vi "Create Resources.vi"(0 "io resources":T1={"address"="SRAM\\Address", "read"="SRAM\\Read", "input valid"="SRAM\\Input Valid", "write data"="SRAM\\Write Data", "read data"="SRAM\\Read Data", "read data valid"="SRAM\\Read Data Valid", "ready for input"="SRAM\\Ready for Input"}) -> (4 "sram resources":T2={"io resources"={"address"="SRAM\\Address", "read"="SRAM\\Read", "input valid"="SRAM\\Input Valid", "write data"="SRAM\\Write Data", "read data"="SRAM\\Read Data", "read data valid"="SRAM\\Read Data Valid", "ready for input"="SRAM\\Ready for Input"}})   [LabVIEW 2011, in "niRFRIO SRAM 1.0.0 FPGA.lvlib"]
uses:
  <instrlib>/RF-RIO/SRAM/1.0.0/FPGA/niRFRIO SRAM 1.0.0 FPGA.lvlib
  <instrlib>/RF-RIO/SRAM/1.0.0/FPGA/Public/Resources.ctl
  <instrlib>/RF-RIO/SRAM/1.0.0/FPGA/Public/IO Resources.ctl
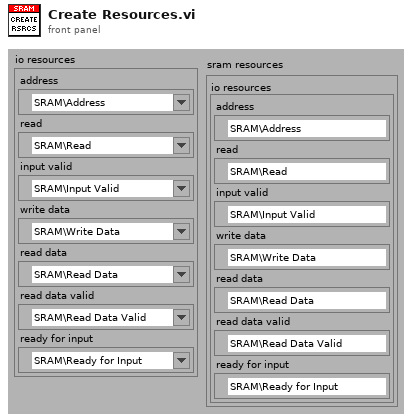
[diagram p1: front panel]
types:
  T1 = typedef "niRFRIO SRAM 1.0.0 FPGA.lvlib/IO Resources.ctl" = cluster{"address":refnum<k21>, "read":refnum<k21>, "input valid":refnum<k21>, "write data":refnum<k21>, "read data":refnum<k21>, "read data valid":refnum<k21>, "ready for input":refnum<k21>}
  T2 = typedef "niRFRIO SRAM 1.0.0 FPGA.lvlib/Resources.ctl" = cluster{"io resources":T1}
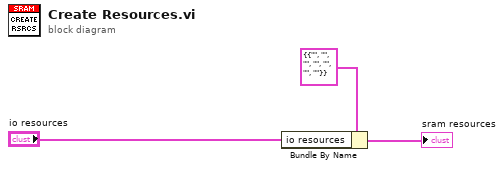
[diagram p0: block diagram]
diagram:
  n1 = Bundle By Name(cluster=T2 {"io resources"={"address"="", "read"="", "input valid"="", "write data"="", "read data"="", "read data valid"="", "ready for input"=""}} ("sram resources"), "io resources"="io resources") -> (→"sram resources":T2)
